vi "Dashboard Main.vi"() -> ()   [LabVIEW 2016]
uses:
  <vilib>/Utility/miscctls.llb/LVRowAndColumnTypeDef.ctl
  <vilib>/event_ctls.llb/eventvkey.ctl
  <vilib>/Rock Robotics/Network Tables/NT Read Numeric Array.vi
  <vilib>/Rock Robotics/WPI/Dashboard/WPI_DashboardLogging Global.vi
  <vilib>/Instr/_visa.llb/VISA Configure Serial Port (Instr).vi
panel:
  in  "Camera Settings Right":T1={"Frame Rate"=30, "Compression"=30, "Size"=1, "DB Camera Config"=FALSE} {"Frame Rate" scale=1.0..30.0; "Compression" scale=100.0..-1.0; "Size" items=["640x480", "320x240", "160x120"]}
  in  "Camera Name Right":string(combo)="No Camera Selection"
  out "Camera Info":cluster{"Mbps LED":bool, "Mbps":dbl, "fps":dbl} {"fps" format="%#.1g"; "Mbps" format="%#.1g"}
  in  "Camera Settings":T1={"Frame Rate"=30, "Compression"=30, "Size"=1, "DB Camera Config"=FALSE} {"Frame Rate" scale=1.0..30.0; "Compression" scale=100.0..-1.0; "Size" items=["640x480", "320x240", "160x120"]}
  in  "TCP":refnum<k5>
  in  "Rec Mode":enum32{"Stop", "Record", "Playback"}(radio)
  out "Robot IP":string
  out "Image Message":string="Timeout in Camera Communications"
  in  "Dashboard Tab":T2(tab)
  in  "Select Auto":string(combo)="Select Autonomous ..."
  out "NT Connection":bool
  out "MotorChart R":cluster{"Numeric":dbl, "Numeric":dbl}(graph)
  out "MotorChart L":cluster{"Numeric":dbl, "Numeric":dbl}(graph)
  out "MotorSliders R":cluster{"MotorSlide1":dbl, "MotorSlide2":dbl} {"MotorSlide2" scale=-1.0..1.0 scale format="%#_2e"; "MotorSlide1" scale=-1.0..1.0 scale format="%#_2e"}
  out "MotorSliders L":cluster{"MotorSlide1":dbl, "MotorSlide2":dbl} {"MotorSlide2" scale=-1.0..1.0 scale format="%#_2e"; "MotorSlide1" scale=-1.0..1.0 scale format="%#_2e"}
  out "Gyro":dbl(knob) scale=0.0..360.0
  out "JS1 Z":dbl(slide) scale=-1.0..1.0 scale format="%#_2e"
  out "JS1 Graph":cluster{"X":dbl, "Y":dbl}[](graph)
  out "JS1 Buttons":T3
  out "JS2 Z":dbl(slide) scale=-1.0..1.0 scale format="%#_2e"
  out "JS2 Graph":cluster{"X":dbl, "Y":dbl}[](graph)
  out "JS2 Buttons":T3
  out "Mode":T4(ring)=enum."Auto Disabled"
  out "read buffer":string
  out "Camera Image Right":T5(plugin-control)
  in  "DB/String 9":string
  in  "DB/String 8":string
  in  "DB/String 7":string
  in  "DB/String 6":string
  in  "DB/String 5":string
  in  "DB/String 4":string
  in  "DB/String 3":string
  in  "DB/String 2":string
  in  "DB/String 1":string
  in  "DB/String 0":string
  in  "DB/Slider 0":dbl(slide) scale=0.0..5.0
  in  "DB/Slider 1":dbl(slide) scale=0.0..5.0
  in  "DB/Slider 2":dbl(slide) scale=0.0..5.0
  in  "DB/Slider 3":dbl(slide) scale=0.0..5.0
  out "DB/LED 3":bool
  out "DB/LED 2":bool
  out "DB/LED 1":bool
  out "DB/LED 0":bool
  in  "DB/Button 3":bool
  in  "DB/Button 2":bool
  in  "DB/Button 1":bool
  in  "DB/Button 0":bool caption="New Name"
  in  "Test Slider":dbl(slide) scale=0.0..100.0 scale format="%#_3g"
  in  "On/Off":bool caption="Solenoid"
  in  "Test Name":u16(ring) items=["Select the test to run..."]
  in  "Test Tree":string(tree)
  in  "Motor":cluster{"Value":dbl, "Enable":bool} {"Value" scale=-1.0..1.0 scale format="%#_3g"}
  out "Progress":T6 {"Test Progress" scale=0.0..100.0}
  in  "Rev/Fwd":cluster{"Forward":bool, "Reverse":bool}
  in  "Test Ring":u16(ring) items=["Monochrome", "Color"]
  out "Cmd Status":string
  in  "Execute Command":bool
  in  "Command Params":string[][](table)
  in  "Command Selection":i32(listbox)
  in  "CheckList":i32(listbox)
  out "Tree":string(tree)
  out "Camera Image":T5(plugin-control)
  out "Background":bool
  in  "Camera Name":string(combo)="No Camera Selection"
  # "HW"
  # "HW"
  # "Joysticks"
  # "Drive Motors"
  # "Front"
  # "Right"
  # "Left"
  # "Back"
  # "This tab is a great place for autonomous settings and robot-specific values.\nPlace controls and indicators inside this tab and match name to\nDashboard Variables on robot. You can also delete this comment."
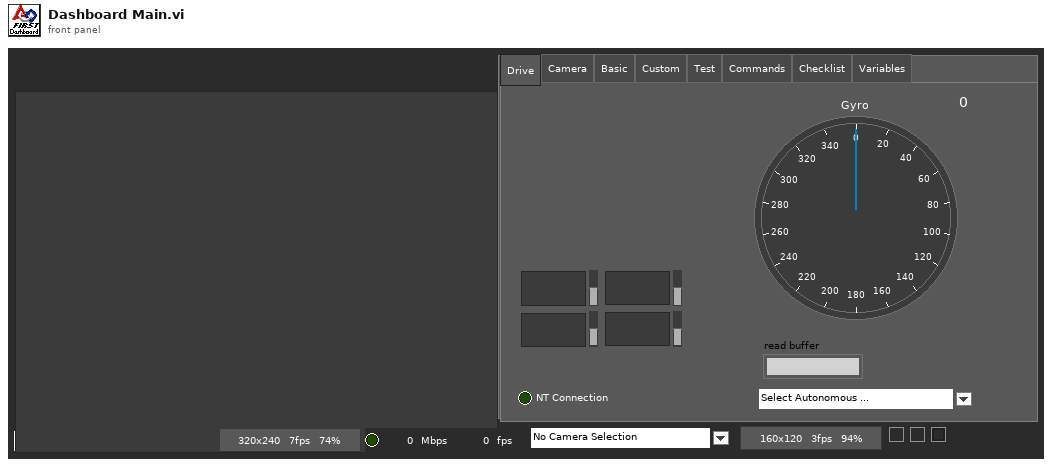
[diagram p1: front panel]
types:
  T1 = cluster{"Frame Rate":i32, "Compression":i32, "Size":u16, "DB Camera Config":bool}
  T2 = enum32{"Drive", "Camera", "Basic", "Custom", "Test", "Commands", "Checklist", "Variables"}
  T3 = cluster{bool, bool, bool, bool, bool, bool, bool, bool, bool, bool, bool, bool}
  T4 = enum8{"Tele-Op Disabled", "Tele-Op Enabled", "Auto Disabled", "Auto Enabled", "Test Disabled", "Test Enabled", "Disconnected", "No Code", "E-Stop"}
  T5 = typedef "IMAQ Image.ctl" = refnum<image>
  T6 = cluster{"Test Progress":u8, "Test Progress Text":string}
  T7 = typedef "Image Type" = u32
  T8 = cluster{"IDs":cluster{"RPC field ID":u16, "Unique ID":u16}, "String":string}
  T9 = enum32{"Drive", "Basic", "Custom", "Test", "Checklist", "Variables"}
  T10 = cluster{"Error Strings":string, "Disable Counts":cluster{u16, u16}, "Rail Faults":cluster{u16, u16, u16}, "Robot IP":string, "DB Mode":u8, "Event Info":cluster{"Name":string, "Type":u8, "Number":u16, "Replay":u8}}
  T11 = cluster{"Storage":cluster{"Disk Free":u64, "RAM Block":u32, "RAM free":u32}, "CPU Utilization":cluster{"CPU % ISR":sgl, "CPU % Time Crit":sgl, "CPU % Timed Str":sgl, "CPU % High":sgl, "CPU % Above":sgl, "CPU % Normal":sgl, "CPU % Low":sgl}, "CAN":cluster{"% Bus Utilization":sgl, "Bus Off Cnt":u32, "TX_FIFO Full Cnt":u32, "Receive Error Cnt":u8, "Transmit Error Cnt":u8}, "HID":cluster{"HID Outputs":u32, "Rumble Low":u16, "Rumble High":u16}[]}
  T12 = cluster{"Status bits":cluster{"Test Mode":bool, "Autonomous":bool, "Enabled":bool, "Code Start":bool, "Brownout":bool, "Reserved 2":bool, "Reserved 3":bool, "E-Stop":bool}, "Code Trace":cluster{"Disabled":bool, "TeleOp":bool, "Auto":bool, "Test":bool}, "Controller Type":enum16{"unknown", "cRIO", "roboRio"}, "Code?":enum16{"unknown", "noCode", "code"}, "Battery V":dbl}
  T13 = cluster{"Control Bits":cluster{"TestMode":bool, "Autonomous":bool, "Enabled":bool, "FMS Present":bool, bool, bool, bool, "E-Stop":bool}, "Team Station ":u8, "Countdown":sgl, "Joystick Values":cluster{"Axes":dbl[], "Buttons":bool[], "POVs":i16[]}[]}
  T14 = cluster{"Axes":dbl[], "Buttons":bool[], "POVs":i16[]}[]
  T15 = cluster{"Axes":dbl[], "Buttons":bool[], "POVs":i16[]}
  T16 = cluster{"Buttons[0]":bool, "Buttons[1]":bool, "Buttons[2]":bool, "Buttons[3]":bool, "Buttons[4]":bool, "Buttons[5]":bool, "Buttons[6]":bool, "Buttons[7]":bool, "Buttons[8]":bool, "Buttons[9]":bool, "Buttons[10]":bool, "Buttons[11]":bool}
  T17 = cluster{"Camera Image":refnum<vi>, "Dashboard Tab":refnum<vi>, "Background":refnum<vi>, "Rec Mode":refnum<vi>, "Test Slider":refnum<vi>, "On/Off ":refnum<vi>, "Test Ring":refnum<vi>, "Rev/Fwd":refnum<vi>, "Test Name":refnum<vi>, "Motor":refnum<vi>, "Progress":refnum<vi>, "CheckList":refnum<vi>, "Tree":refnum<vi>, "Test Tree":refnum<vi>, "Command Params":refnum<vi>, "Command Selection":refnum<vi>, "Execute Command":refnum<vi>, "Cmd Status":refnum<vi>, "Camera Settings":refnum<vi>, "Camera Name":refnum<vi>, "Camera Info":refnum<vi>, "Camera Settings Right":refnum<vi>, "Camera Name Right":refnum<vi>, "Camera Image Right":refnum<vi>}
  T18 = cluster{"Operation":enum16{"Update", "Clear"}, "Color Box":u32}[]
  T19 = typedef "eventvkey.ctl" = enum16{"ASCII", "Enter", "Return", "Shift", "Ctrl", "Alt", "Cmd", "Opt", "Caps", "NumLock", "Clear", "Break", "Up", "Down", "Left", "Right", "Insert", "Delete", "Home", "End", "PageUp", "PageDown", "Escape", "Help", "Pause", "ScrollLock", "F1", "F2", "F3", "F4", "F5", "F6", "F7", "F8", "F9", "F10", "F11", "F12", "F13", "F14", "F15", "F16", "F17", "F18", "F19", "F20", "F21", "F22", "F23", "F24", "Play", "VolumeUp", "VolumeDown", "Mute", "Two Byte Char"}
  T20 = cluster{"Image Size":bool, "Image Type":bool, "Pixel Value":bool, "ROI Information":bool, "Zoom Factor":bool}
  T21 = cluster{"Operation":enum16{"Update", "Clear"}, "Color Box":u32}
  T22 = typedef "LVRowAndColumnTypeDef.ctl" = cluster{"Row":i32, "Column":i32}
  T23 = cluster{"Shift":bool, "Ctrl":bool, "Alt":bool, "Cmd":bool, "Opt":bool}
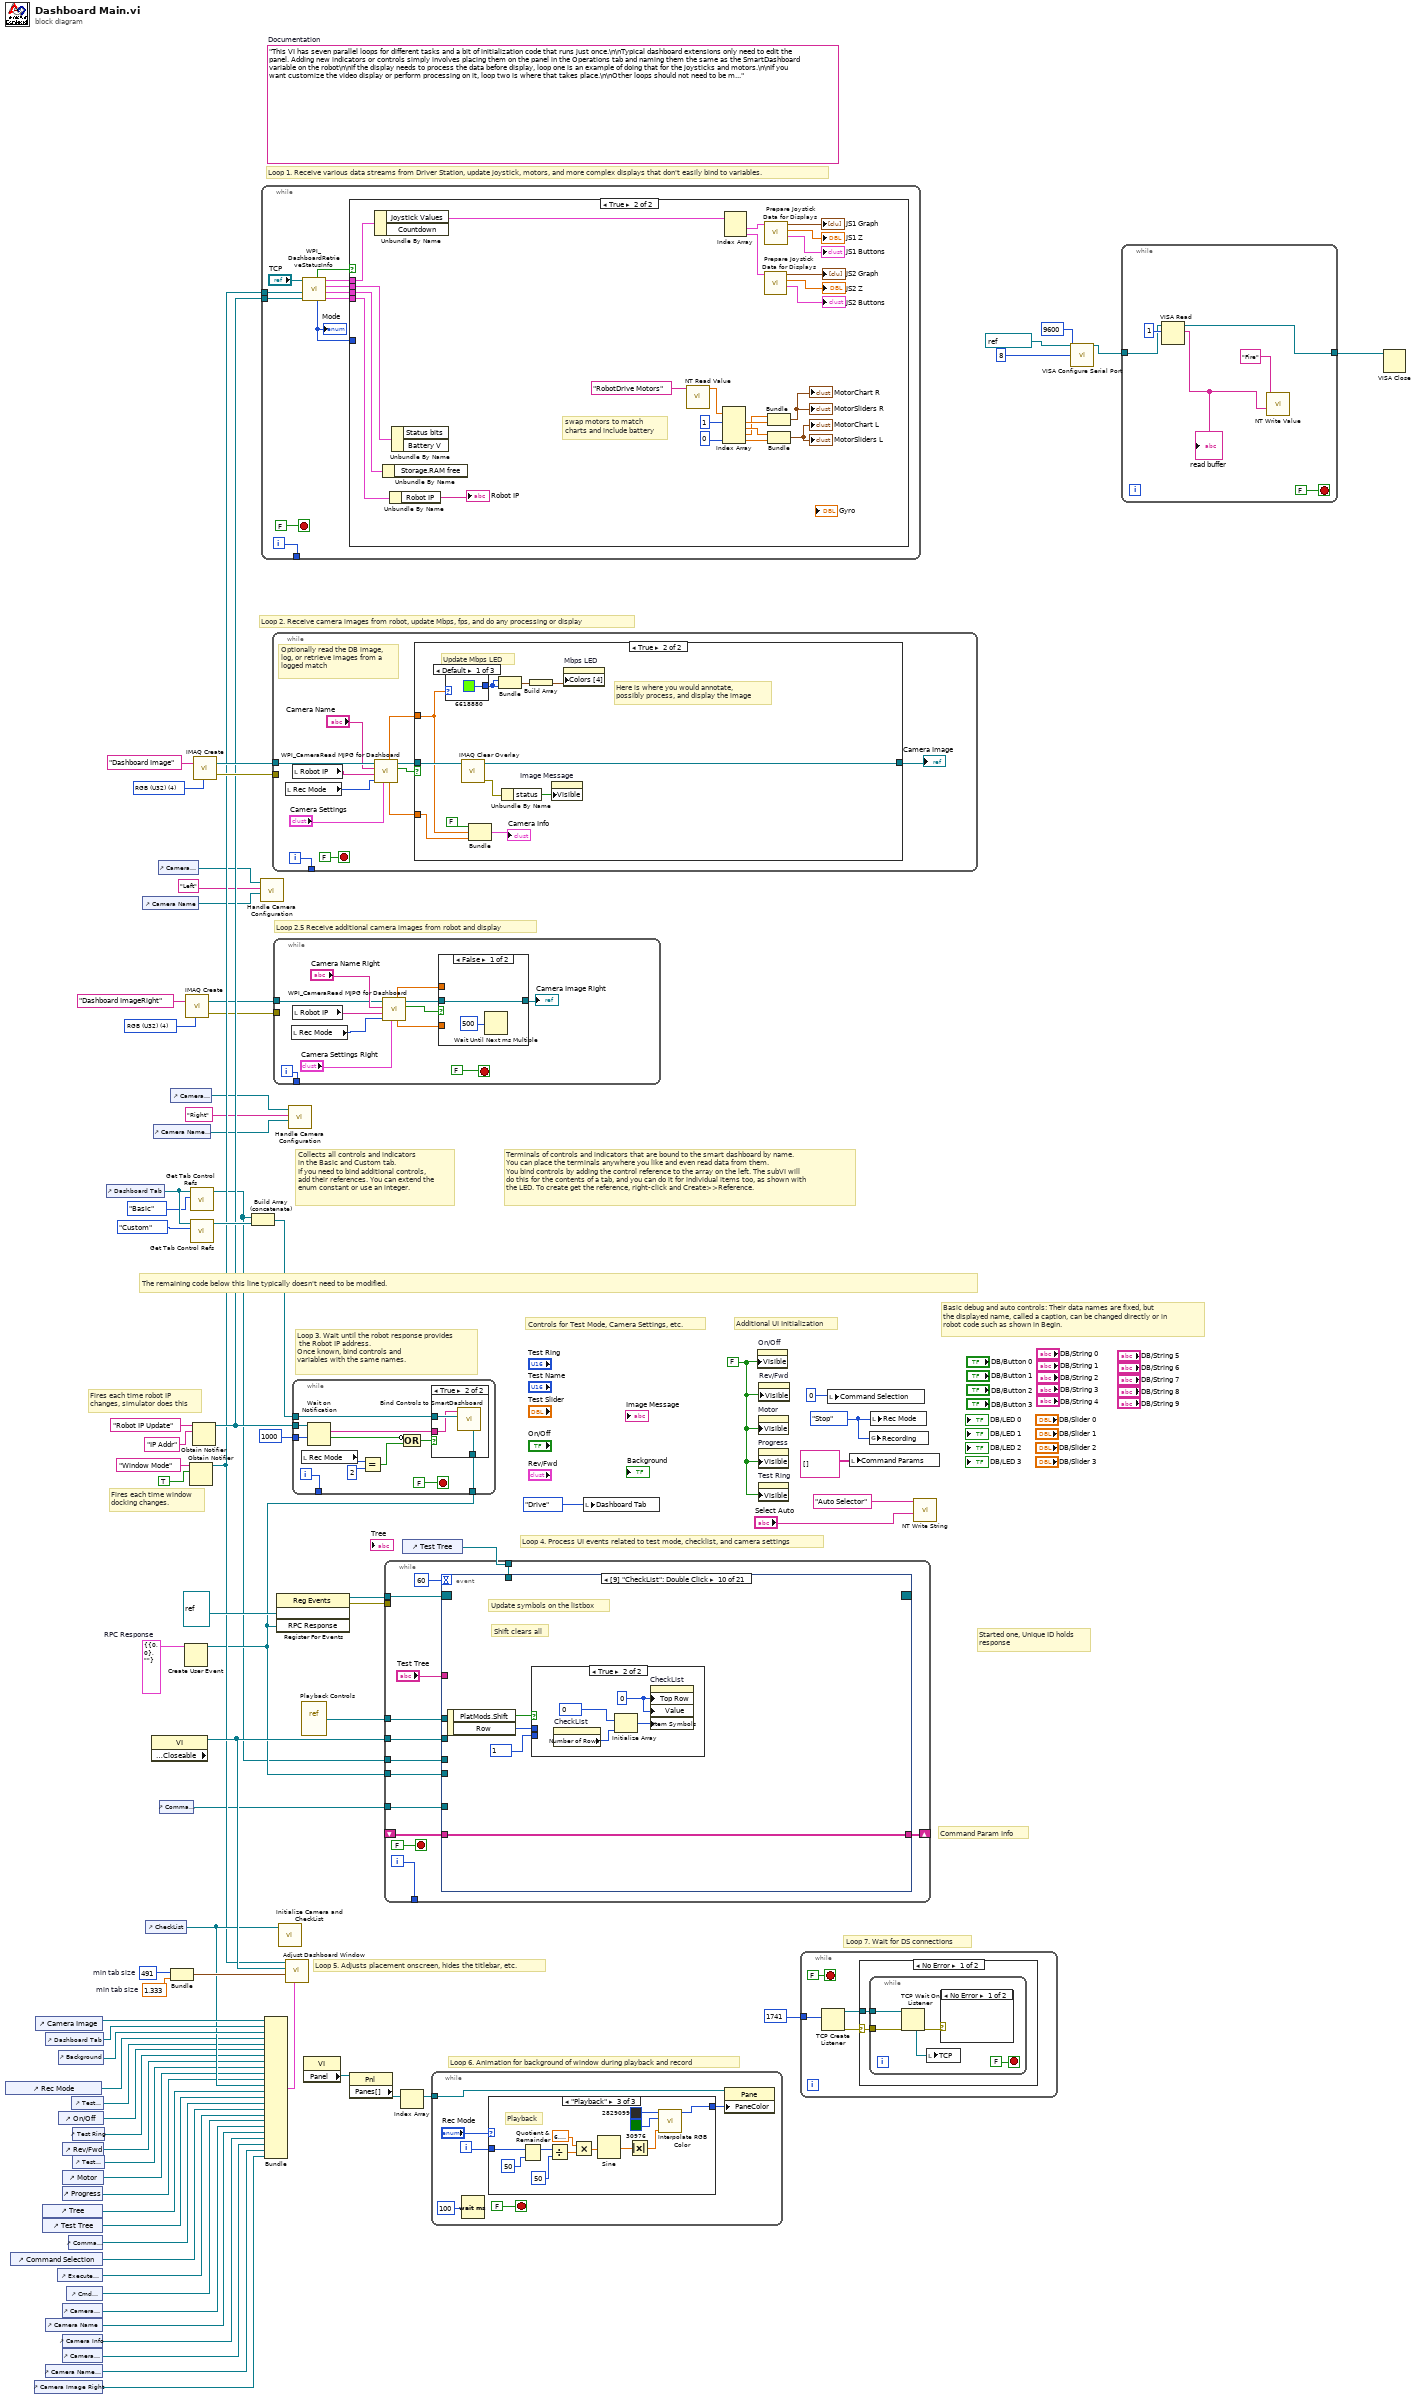
[diagram p0: block diagram]
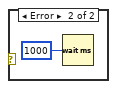
[diagram p3: hidden frame]
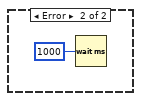
[diagram p4: hidden frame]
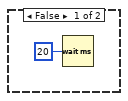
[diagram p5: hidden frame]
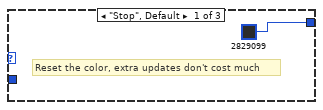
[diagram p6: hidden frame]
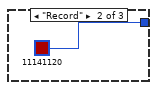
[diagram p7: hidden frame]
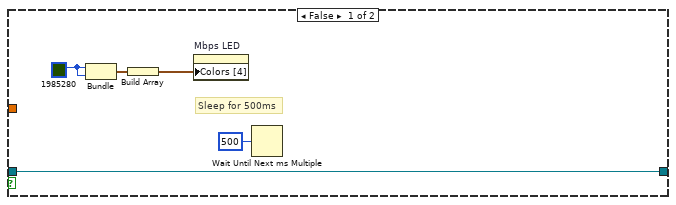
[diagram p9: hidden frame]
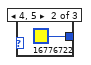
[diagram p10: hidden frame]
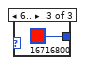
[diagram p11: hidden frame]
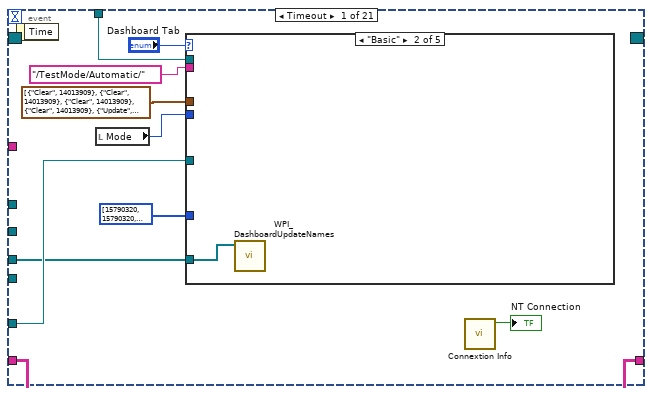
[diagram p12: hidden frame]
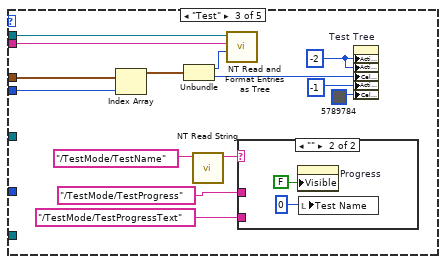
[diagram p14: hidden frame]
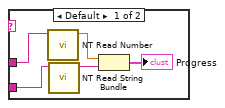
[diagram p15: hidden frame]
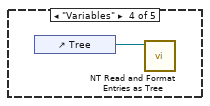
[diagram p16: hidden frame]
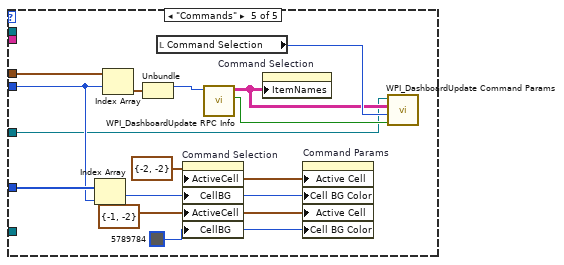
[diagram p17: hidden frame]
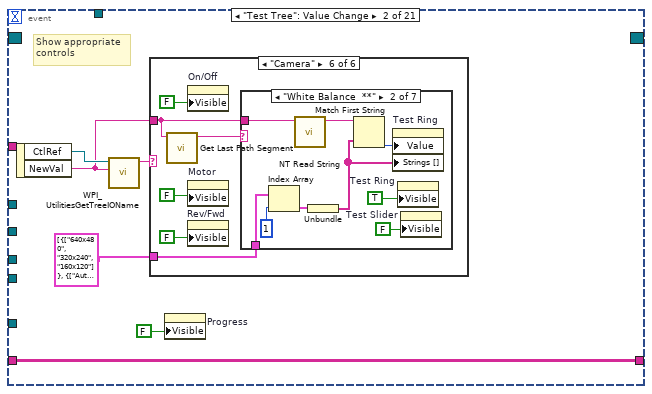
[diagram p18: hidden frame]
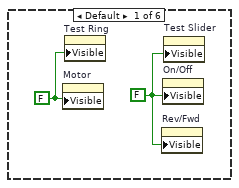
[diagram p19: hidden frame]
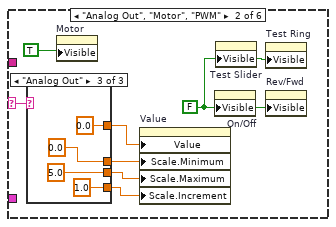
[diagram p20: hidden frame]
diagram:
  w15 = T7 4 items=["Grayscale (U8)", "Grayscale (I16)", "Grayscale (SGL)", "Complex (CSG)", "RGB (U32)", "HSL (U32)", "RGB (U64)"] ("Image Type")
  w31 = T8 {"IDs"={"RPC field ID"=0, "Unique ID"=0}, "String"=""}  # RPC Response
  w56 = 491  # min tab size
  w55 = 1.333  # min tab size
  w63 = enum32{"Stop", "Record", "Playback"}."Stop" ("Rec Mode")
  w38 = FALSE ("Visible")
  (unwired) "This VI has seven parallel loops for different tasks and a bit of initialization code that runs just once.\n\nTypical dashboard extensions only need to edit the panel. Adding new indicators or controls simply involves placing them on the panel in the Operations tab and naming them the same as the SmartDashboard variable on the robot\n\nIf the display needs to process the data before display, loop one is an example of doing that for the joysticks and motors.\n\nIf you want customize the video display or perform processing on it, loop two is where that takes place.\n\nOther loops should not need to be modified. They are pretty standard, and document the task they perform."  # Documentation
  w80 = T7 4 items=["Grayscale (U8)", "Grayscale (I16)", "Grayscale (SGL)", "Complex (CSG)", "RGB (U32)", "HSL (U32)", "RGB (U64)"] ("Image Type")
  # "Loop 2.5 Receive additional camera images from robot and display"
  # "Command Param Info"
  # "Started one, Unique ID holds\nresponse"
  # "Loop 7. Wait for DS connections"
  # "Basic debug and auto controls: Their data names are fixed, but\nthe displayed name, called a caption, can be changed directly or in\nrobot code such as shown in Begin."
  # "Controls for Test Mode, Camera Settings, etc."
  # "Additional UI Initialization"
  # "Loop 6. Animation for background of window during playback and record"
  # "Fires each time robot IP\nchanges, simulator does this"
  # "Fires each time window\ndocking changes."
  # "Collects all controls and indicators\nin the Basic and Custom tab.\nIf you need to bind additional controls,\nadd their references. You can extend the\nenum constant or use an integer."
  # "The remaining code below this line typically doesn't need to be modified."
  # "Loop 4. Process UI events related to test mode, checklist, and camera settings"
  # "Terminals of controls and indicators that are bound to the smart dashboard by name.\nYou can place the terminals anywhere you like and even read data from them.\nYou bind controls by adding the control reference to the array on the left. The subVI will\ndo this for the contents of a tab, and you can do it for individual items too, as shown with\nthe LED. To create get the reference, right-click and Create>>Reference."
  # "Loop 3. Wait until the robot response provides\n the Robot IP address.\nOnce known, bind controls and\nvariables with the same names."
  # "Loop 5. Adjusts placement onscreen, hides the titlebar, etc."
  # "Loop 1. Receive various data streams from Driver Station, update joystick, motors, and more complex displays that don't easily bind to variables."
  # "Loop 2. Receive camera images from robot, update Mbps, fps, and do any processing or display"
  n1 = control-ref of="Rec Mode"() -> (w44:refnum<vi>)
  n2 = control-ref of="Command Selection"() -> (w30:refnum<vi>)
  n3 = control-ref of="Camera Image Right"() -> (w6:refnum<vi>)
  n4 = control-ref of="Camera Image"() -> (w58:refnum<vi>)
  n5 = control-ref of="Tree"() -> (w48:refnum<vi>)
  n6 = control-ref of="Test Tree"() -> (w47:refnum<vi>)
  n7 = control-ref of="Dashboard Tab"() -> (w57:refnum<vi>)
  n8 = control-ref of="Camera Name"() -> (w21:refnum<vi>)
  n9 = control-ref of="Camera Name Right"() -> (w7:refnum<vi>)
  n10 = control-ref of="Execute Command"() -> (w32:refnum<vi>)
  n11 = control-ref of="Background"() -> (w53:refnum<vi>)
  n12 = control-ref of="On/Off"() -> (w42:refnum<vi>)
  n13 = control-ref of="Progress"() -> (w39:refnum<vi>)
  n14 = control-ref of="Camera Settings"() -> (w22:refnum<vi>)
  n15 = control-ref of="Camera Info"() -> (w20:refnum<vi>)
  n16 = control-ref of="Camera Settings Right"() -> (w8:refnum<vi>)
  n17 = control-ref of="Rev/Fwd"() -> (w40:refnum<vi>)
  n18 = control-ref of="Motor"() -> (w45:refnum<vi>)
  n19 = control-ref of="Cmd Status"() -> (w26:refnum<vi>)
  n20 = control-ref of="Command Params"() -> (w33:refnum<vi>)
  n21 = control-ref of="Test Slider"() -> (w43:refnum<vi>)
  n22 = control-ref of="Test Ring"() -> (w41:refnum<vi>)
  n23 = control-ref of="Test Name"() -> (w46:refnum<vi>)
  n24 = control-ref of="Dashboard Tab"() -> (w61:refnum<vi>)
  n25 = control-ref of="Camera Name"() -> (w23:refnum<vi>)
  n26 = control-ref of="CheckList"() -> (w49:refnum<vi>)
  n27 = property class="VI" props=["Front Panel.Closeable"]() -> (reference out=w62:refnum<vi>)  [unwired: 2 in, 2 out]
  n28 = control-ref of="Camera Name Right"() -> (w11:refnum<vi>)
  n29 = control-ref of="Camera Settings"() -> (w24:refnum<vi>)
  n30 = control-ref of="Command Params"() -> (w25:refnum<vi>)
  n31 = control-ref of="Camera Settings Right"() -> (w12:refnum<vi>)
  n32 = Bundle("min tab size"=w56, "min tab size"=w55) -> (w54:cluster{"min tab size":i32, "min tab size":dbl})  [unwired: 1 in]
  n33 = Create User Event(user event datatype=w31) -> (user event=w27:refnum<user-event>)  [unwired: 1 in, 1 out]
  n34 = call "IMAQ Create"("Image Name"="Dashboard ImageRight", "Image Type"=w15) -> ("New Image"=w14:T5, "error out"=w13:errorcluster)  [unwired: 2 in, 1 out]
  n35 = Obtain Notifier(name (unnamed)="Window Mode", notification data type=TRUE) -> (notifier out=w36:refnum<notifier>)  [unwired: 2 in, 2 out]
  n36 = call <vilib>:"Get Tab Control Refs.vi"("Page Index"=T9."Basic" ("Dashboard Tab"), "TabControl in"=w61) -> ("ControlsOnPage"=w19:refnum<vi>[])  [unwired: 9 in]
  n37 = call <vilib>:"Get Tab Control Refs.vi"("Page Index"=T9."Custom" ("Dashboard Tab"), "TabControl in"=w61) -> ("ControlsOnPage"=w60:refnum<vi>[])  [unwired: 9 in]
  n38 = Obtain Notifier(name (unnamed)="Robot IP Update", notification data type="IP Addr" ("name (unnamed)")) -> (notifier out=w37:refnum<notifier>)  [unwired: 2 in, 2 out]
  n39 = call "IMAQ Create"("Image Name"="Dashboard Image", "Image Type"=w80) -> ("New Image"=w78:T5, "error out"=w77:errorcluster)  [unwired: 2 in, 1 out]
  n40 = Build Array (concatenate)(w19, w60) -> (w59:refnum<vi>[])
  n41 = call "Handle Camera Configuration.vi"("CameraNameRef"=w23, "Camera File Name"="Left", "ClusterRef"=w24) -> ()  [unwired: 9 in]
  n42 = while {
    tunnel: [w90] -> _
    tunnel: w37 -> [w84]
    tunnel: w36 -> [w81]
    i -> [w90]
    stop <- FALSE stop-if-true
    n43 = call <vilib>:"WPI_DashboardRetrieveStatusInfo.vi"("Binding Refnum"=w84, "Window Mode Notifier"=w81, "TCP Cnx"="TCP") -> ("Power and Errors"=w85:T10, "Robot Metrics"=w88:T11, "Status Info"=w89:T12, "Control Info"=w86:T13, "Robot Mode"=w83:T4, "Process?"=w87:bool)  [unwired: 3 in]
    "Mode" <- w83
    n44 = case shown="True" w87 {
      tunnel: w89 -> [_ w116]
      tunnel: w88 -> [_ w115]
      tunnel: w86 -> [_ w114]
      tunnel: w85 -> [_ w113]
      tunnel: w83 -> [_ _]
      frame False {
        n45 = Wait (ms)(milliseconds to wait=u32 20) -> ()  [unwired: 1 out]
      }
      frame True {
        # "swap motors to match\ncharts and include battery"
        n46 = Unbundle By Name(w114) -> ("Joystick Values"=w104:T14)  [unwired: 1 out]
        n47 = Unbundle By Name(w115) -> ()  [unwired: 1 out]
        n48 = Unbundle By Name(w113) -> ("Robot IP"=→"Robot IP":string)
        n49 = Unbundle By Name(w116) -> ()  [unwired: 2 out]
        n50 = call-poly <vilib>:"NT Read Value.vi"("Name"="RobotDrive Motors") -> ("Numeric Array"=w94:dbl[])  [unwired: 9 in, 1 out]
        n51 = Index Array(array=w94, index #1=1, index #4=0) -> (element #1=w108:dbl, element #2=w109:dbl, element #3=w107:dbl, element #4=w112:dbl)  [unwired: 2 in]
        n52 = Index Array(array=w104) -> (element #1=w103:T15, element #2=w99:T15)  [unwired: 2 in]
        n53 = call "Prepare Joystick Data for Displays.vi"("Joystick Values"=w99) -> ("Buttons"=→"JS2 Buttons":T16, "Z Axis"=→"JS2 Z":dbl, "Cartesian Data"=→"JS2 Graph":cluster{"X axis":dbl, "X axis":dbl}[])  [unwired: 8 in]
        n54 = call "Prepare Joystick Data for Displays.vi"("Joystick Values"=w103) -> ("Buttons"=→"JS1 Buttons":T16, "Z Axis"=→"JS1 Z":dbl, "Cartesian Data"=→"JS1 Graph":cluster{"X axis":dbl, "X axis":dbl}[])  [unwired: 8 in]
        n55 = Bundle("Numeric"=w107, "Numeric"=w108) -> (→"MotorChart R" →"MotorSliders R":cluster{"Numeric":dbl, "Numeric":dbl})  [unwired: 1 in]
        n56 = Bundle("Numeric"=w109, "Numeric"=w112) -> (→"MotorChart L" →"MotorSliders L":cluster{"Numeric":dbl, "Numeric":dbl})  [unwired: 1 in]
      }
    }
  }
  n57 = Bundle("Camera Image"=w58, "Dashboard Tab"=w57, "Background"=w53, "Rec Mode"=w44, "Test Slider"=w43, "On/Off"=w42, "Test Ring"=w41, "Rev/Fwd"=w40, "Test Name"=w46, "Motor"=w45, "Progress"=w39, "CheckList"=w49, "Tree"=w48, "Test Tree"=w47, "Command Params"=w33, "Command Selection"=w30, "Execute Command"=w32, "Cmd Status"=w26, "Camera Settings"=w22, "Camera Name"=w21, "Camera Info"=w20, "Camera Settings Right"=w8, "Camera Name Right"=w7, "Camera Image Right"=w6) -> (w50:T17)  [unwired: 1 in]
  n58 = while {
    tunnel: w78 -> [w126]
    tunnel: w77 -> [_]
    tunnel: [w127] -> _
    i -> [w127]
    stop <- FALSE stop-if-true
    # "Optionally read the DB image,\nlog, or retrieve images from a\nlogged match"
    n59 = local read "Rec Mode"() -> (w122:enum32{"Stop", "Record", "Playback"})
    n60 = local read "Robot IP"() -> (w121:string)
    n61 = call <vilib>:"WPI_CameraRead MJPG for Dashboard.vi"("Camera Settings"="Camera Settings", "Rec Mode"=w122, "Robot IP"=w121, "Camera Name"="Camera Name", "Refnum in"=w126) -> ("Active"=w124:bool, "Refnum out"=w125:T5, "FPS"=w123:dbl, "Bandwidth (Mbps)"=w120:dbl)  [unwired: 3 in]
    n62 = case shown="True" w124 {
      tunnel: w125 -> [w129 w140]
      tunnel: w120 -> [_ w137]
      tunnel: w123 -> [_ w138]
      tunnel: [w129 w134] -> w117
      frame False {
        w131 = u32 1985280 ("Color Box")
        # "Sleep for 500ms"
        n63 = Bundle("Color Box"=w131, "Color Box"=w131) -> (w132:cluster{"Color Box":u32, "Color Box":u32})  [unwired: 1 out]
        n64 = Build Array(w132) -> (w130:cluster{"Color Box":u32, "Color Box":u32}[])
        n65 = property on="Mbps LED" class="Bool (strict)"("Colors [4]"=w130) -> ()  [unwired: 2 in, 2 out]
        n66 = Wait Until Next ms Multiple(millisecond multiple=u32 500) -> ()  [unwired: 1 out]
      }
      frame True {
        # "Here is where you would annotate,\npossibly process, and display the image"
        # "Update Mbps LED"
        n67 = case shown="Default" w137 {
          tunnel: [u32 6618880 ("Color Box") u32 16776722 ("Color Box") u32 16716800 ("Color Box")] -> w141
          frame Default {
          }
          frame 4, 5 {
          }
          frame 6.. {
          }
        }
        n68 = call "IMAQ Clear Overlay"("Image"=w140) -> ("error out"=w143:errorcluster, "Image Out"=w134:T5)  [unwired: 2 in, 7 out]
        n69 = Bundle(FALSE, "Bandwidth (Mbps)"=w137, "FPS"=w138) -> (→"Camera Info":cluster{bool, "Bandwidth (Mbps)":dbl, "FPS":dbl})  [unwired: 1 in]
        n70 = Bundle("Color Box"=w141, "Color Box"=w141) -> (w142:cluster{"Color Box":u32, "Color Box":u32})  [unwired: 1 out]
        n71 = Unbundle By Name(w143) -> ("status"=w144:bool)
        n72 = Build Array(w142) -> (w139:cluster{"Color Box":u32, "Color Box":u32}[])
        n73 = property on="Image Message" class="Str"("Visible"=w144) -> ()  [unwired: 2 in, 2 out]
        n74 = property on="Mbps LED" class="Bool (strict)"("Colors [4]"=w139) -> ()  [unwired: 2 in, 2 out]
      }
    }
    "Camera Image" <- w117
  }
  n75 = while {
    tunnel: w14 -> [w158]
    tunnel: w13 -> [_]
    tunnel: [w152] -> _
    i -> [w152]
    stop <- FALSE stop-if-true
    n76 = local read "Rec Mode"() -> (w156:enum32{"Stop", "Record", "Playback"})
    n77 = local read "Robot IP"() -> (w157:string)
    n78 = call <vilib>:"WPI_CameraRead MJPG for Dashboard.vi"("Camera Settings"="Camera Settings Right", "Rec Mode"=w156, "Robot IP"=w157, "Camera Name"="Camera Name Right", "Refnum in"=w158) -> ("Active"=w151:bool, "Refnum out"=w154:T5, "FPS"=w149:dbl, "Bandwidth (Mbps)"=w150:dbl)  [unwired: 3 in]
    n79 = case shown="False" w151 {
      tunnel: w154 -> [w160 w162]
      tunnel: w150 -> [_ _]
      tunnel: w149 -> [_ _]
      tunnel: [w160 w162] -> w148
      frame False {
        n80 = Wait Until Next ms Multiple(millisecond multiple=u32 500) -> ()  [unwired: 1 out]
      }
      frame True {
      }
    }
    "Camera Image Right" <- w148
  }
  n81 = register-events(refnum<vi> refnum, w27) -> (reference out=w67:refnum<event-registration>, error out=w66:errorcluster)  [unwired: 2 in]
  n82 = call "Initialize Camera and CheckList.vi"("ListBox in"=w49) -> ()  [unwired: 11 in]
  n83 = call "Adjust Dashboard Window.vi"("Sizing Refnums"=w50, "Size Constraints"=w54, "VI"=w62, "WIn Mode"=w36) -> ()  [unwired: 8 in]
  n84 = call "Handle Camera Configuration.vi"("CameraNameRef"=w11, "Camera File Name"="Right", "ClusterRef"=w12) -> ()  [unwired: 9 in]
  n85 = while {
    tunnel: w59 -> [w174]
    tunnel: w37 -> [w172]
    tunnel: [w170] -> _
    tunnel: u32 1000 ("milliseconds to wait") -> [w169]
    tunnel: w27 -> [w163]
    i -> [w170]
    stop <- FALSE stop-if-true
    n86 = local read "Rec Mode"() -> (w165:enum32{"Stop", "Record", "Playback"})
    n87 = Wait on Notification(notifier=w172, timeout in ms (-1)=w169) -> (notification=w171:string, timed out?=w167:bool)  [unwired: 2 in, 2 out]
    n88 = Equal?(x=w165, y=u16 2 ("Rec Mode")) -> (x = y?=w166:bool)
    n89 = Compound Arithmetic op=OR(invert w167, w166) -> (w168:bool)
    n90 = case shown="True" w168 {
      tunnel: w174 -> [_ w177]
      tunnel: w171 -> [_ w176]
      tunnel: w163 -> [_ w175]
      frame False {
      }
      frame True {
        n91 = call <vilib>:"Bind Controls to SmartDashboard.vi"("RPC ref"=w175, "Bound Control Refs"=w177, "Server IP Address"=w176) -> ()  [unwired: 9 in]
      }
    }
  }
  n92 = vi-ref "Playback Controls.vi"() -> (w68:refnum<vi>)
  n93 = property class="VI"() -> ("Panel"=w70:refnum<vi>)  [unwired: 2 in, 2 out]
  n94 = property class="Pnl"(reference=w70) -> ("Panes[]"=w71:refnum<vi>[])  [unwired: 1 in, 2 out]
  n95 = Index Array(array=w71) -> (element=w69:refnum<vi>)  [unwired: 1 in]
  n96 = control-ref of="Test Tree"() -> (w72:refnum<vi>)
  n97 = while {
    tunnel: [w187] -> _
    tunnel: w72 -> [w186]
    tunnel: w68 -> [w185]
    tunnel: w67 -> [w184]
    tunnel: w66 -> [_]
    tunnel: w62 -> [w183]
    tunnel: w27 -> [w182]
    tunnel: w25 -> [w181]
    shift-right: [w180] -> _
    shift-left: _ -> [w179]
    tunnel: w19 -> [w178]
    i -> [w187]
    stop <- FALSE stop-if-true
    n98 = event shown="[9] \"CheckList\": Double Click" {
      selector: w184 -> [_ _ _ _ _ _ _ _ _ _ _ _ _ _ _ _ _ _ _ _ _]
      dyn-events: [_ _ _ _ _ _ _ _ _ _ _ _ _ _ _ _ w443 _ _ _ _] -> _
      timeout: u32 60 ("milliseconds to wait") -> [_ _ _ _ _ _ _ _ _ _ _ _ _ _ _ _ _ _ _ _ _]
      tunnel: w186 -> [w199 _ _ _ _ _ _ _ _ _ _ _ _ _ _ _ _ _ _ _ _]
      tunnel: "Test Tree" -> [_ _ _ _ _ _ _ _ _ _ _ w410 w418 w420 w424 w432 _ _ _ _ _]
      tunnel: w185 -> [_ _ _ _ _ _ _ _ _ _ _ _ _ _ _ _ w445 _ w463 _ _]
      tunnel: w183 -> [_ _ _ _ _ _ _ _ _ _ _ _ _ _ _ _ w441 _ _ _ _]
      tunnel: w182 -> [_ _ _ _ _ _ _ _ _ _ _ _ _ _ _ _ w437 _ _ _ _]
      tunnel: w181 -> [w194 _ _ _ _ _ w361 _ _ _ _ _ _ _ _ _ _ _ _ _ _]
      tunnel: [w193 w238 w340 w345 w354 w358 w359 w368 w378 w385 w397 w409 w416 w419 w423 w431 w436 w458 w460 w464 w475] -> w180
      tunnel: w179 -> [w193 w238 w340 w345 w354 w358 w359 _ _ w385 w397 w409 w416 w419 w423 w431 w436 w458 w460 w464 w475]
      tunnel: w178 -> [w191 _ _ _ _ _ _ _ _ _ _ _ _ _ _ _ _ _ _ _ _]
      event Timeout {
        n99 = event-data() -> ()  [unwired: 1 in, 1 out]
        n100 = local read "Mode"() -> (w196:T4)
        n101 = case shown="\"Basic\"" "Dashboard Tab" {
          tunnel: w199 -> [_ _ w215 _ _]
          tunnel: "/TestMode/Automatic/" ("Name Pattern") -> [_ _ w214 _ _]
          tunnel: T18 [{"Operation"=enum."Clear", "Color Box"=14013909}, {"Operation"=enum."Clear", "Color Box"=14013909}, {"Operation"=enum."Clear", "Color Box"=14013909}, {"Operation"=enum."Clear", "Color Box"=14013909}, {"Operation"=enum."Update", "Color Box"=14013909}, {"Operation"=enum."Update", "Color Box"=16777215}, {"Operation"=enum."Clear", "Color Box"=14013909}, {"Operation"=enum."Clear", "Color Box"=14013909}, {"Operation"=enum."Clear", "Color Box"=14013909}] -> [_ _ w207 _ w231]
          tunnel: w196 -> [_ _ w206 _ w230]
          tunnel: u32[] [15790320, 15790320, 15790320, 15790320, 16777215, 16777215, 15790320, 15790320, 15790320] -> [_ _ _ _ w236]
          tunnel: w194 -> [_ _ _ _ w224]
          tunnel: w191 -> [_ w201 _ _ _]
          frame "Custom", Default {
          }
          frame "Basic" {
            n102 = call <vilib>:"WPI_DashboardUpdateNames.vi"("Controls on Tab"=w201) -> ()  [unwired: 11 in]
          }
          frame "Test" {
            w213 = -2 ("Active Item:Row Number")
            n103 = Index Array(array=w207, index=w206) -> (element=w208:T21)
            n104 = Unbundle(w208) -> ("Operation"=w209:enum16{"Update", "Clear"}, "Color Box"=w210:u32)
            n105 = call <vilib>:"NT Read String.vi"("Name"="/TestMode/TestName") -> ("String"=w204:string)  [unwired: 9 in, 1 out]
            n106 = call <vilib>:"NT Read and Format Entries as Tree.vi"("Operation"=w209, "Name Pattern"=w214, "Tree Refnum"=w215) -> ()  [unwired: 7 in, 2 out]
            n107 = case shown="\"\"" w204 {
              tunnel: "/TestMode/TestProgress" ("Name") -> [w217 _]
              tunnel: "/TestMode/TestProgressText" ("Name") -> [w216 _]
              frame Default {
                n108 = call <vilib>:"NT Read Number.vi"("Name"=w217) -> ("Numeric"=w218:dbl)  [unwired: 9 in, 1 out]
                n109 = call <vilib>:"NT Read String.vi"("Name"=w216) -> ("String"=w219:string)  [unwired: 9 in, 1 out]
                n110 = Bundle("Numeric"=w218, "String"=w219) -> (→"Progress":cluster{"Numeric":dbl, "String":string})  [unwired: 1 in]
              }
              frame "" {
                n111 = property on="Progress" class="Clust (strict)"("Visible"=FALSE) -> ()  [unwired: 2 in, 2 out]
                n112 = local write "Test Name"(u16 0) -> ()
              }
            }
            n113 = property on="Test Tree" class="Tree (strict)"("Active Item Row Number"=w213, "ActiveColNum"=w213, "CellBG"=w210, "Active Item Row Number"=-1 ("Active Item:Row Number"), "CellBG"=u32 5789784 ("Color Box")) -> ()  [unwired: 2 in, 2 out]
          }
          frame "Variables" {
            n114 = control-ref of="Tree"() -> (w223:refnum<vi>)
            n115 = call <vilib>:"NT Read and Format Entries as Tree.vi"("Tree Refnum"=w223) -> ()  [unwired: 9 in, 2 out]
          }
          frame "Commands" {
            w232 = u32 5789784 ("Color Box")
            w233 = T22 {"Row"=-1, "Column"=-2} ("Active Cell:Active Cell")
            w235 = T22 {"Row"=-2, "Column"=-2} ("Active Cell:Active Cell")
            n116 = Index Array(array=w236, index=w230) -> (element=w234:u32)
            n117 = Index Array(array=w231, index=w230) -> (element=w229:T21)
            n118 = Unbundle(w229) -> ("Operation"=w228:enum16{"Update", "Clear"})  [unwired: 1 out]
            n119 = local read "Command Selection"() -> (w227:i32)
            n120 = property on="Command Selection" class="MCListbox (strict)"("ActiveCell"=w235, "CellBG"=w234, "ActiveCell"=w233, "CellBG"=w232) -> ()  [unwired: 2 in, 2 out]
            n121 = call <vilib>:"WPI_DashboardUpdate RPC Info.vi"("Operation"=w228) -> ("update"=w226:bool, "commands"=w225:string[][])  [unwired: 9 in]
            n122 = property on="Command Selection" class="MCListbox (strict)"("ItemNames"=w225) -> ()  [unwired: 2 in, 2 out]
            n123 = property on="Command Params" class="Tbl (strict)"("Active Cell"=w235, "Cell BG Color"=w234, "Active Cell"=w233, "Cell BG Color"=w232) -> ()  [unwired: 2 in, 2 out]
            n124 = call <vilib>:"WPI_DashboardUpdate Command Params.vi"("Update"=w226, "NewVal"=w227, "Commands"=w225, "Param Tbl"=w224) -> ()  [unwired: 7 in, 1 out]
          }
        }
        n125 = call <vilib>:"Connextion Info.vi"() -> ("Connected"=→"NT Connection":bool)  [unwired: 10 in, 1 out]
      }
      event "Test Tree": Value Change {
        # "Show appropriate\ncontrols"
        n126 = event-data() -> ("CtlRef"=w241:refnum<vi>, "NewVal"=w239:string)  [unwired: 1 in]
        n127 = call <vilib>:"WPI_UtilitiesGetTreeIOName.vi"("NewVal"=w239, "TreeControl in"=w241) -> ("I/O Name"=w242:string)  [unwired: 9 in]
        n128 = case shown="\"Camera\"" w242 {
          selector: w242 -> [_ w249 _ w271 w280 _]
          tunnel: w239 -> [_ _ w268 w270 _ w287]
          tunnel: cluster{string[]}[] [{["640x480", "320x240", "160x120"]}, {["Auto", "Fixed indoor", "Fixed outdoor 1", "Fixed outdoor 2", "Fixed fluorescent 1", "Fixed fluorescent 2", "Hold current"]}, {["Auto", "Flicker-free 50 Hz", "Flicker-free 60 Hz", "Hold current"]}, {["None", "Prioritize frame rate", "Prioritize image quality"]}, {["Monochrome", "Color"]}] -> [_ _ _ _ _ w286]
          frame Default {
            w244 = FALSE ("Visible")
            w243 = FALSE ("Visible")
            n129 = property on="Motor" class="Clust (strict)"("Visible"=w243) -> ()  [unwired: 2 in, 2 out]
            n130 = property on="Test Ring" class="Ring (strict)"("Visible"=w243) -> ()  [unwired: 2 in, 2 out]
            n131 = property on="Rev/Fwd" class="Clust (strict)"("Visible"=w244) -> ()  [unwired: 2 in, 2 out]
            n132 = property on="On/Off" class="Bool (strict)"("Visible"=w244) -> ()  [unwired: 2 in, 2 out]
            n133 = property on="Test Slider" class="Slide (strict)"("Visible"=w244) -> ()  [unwired: 2 in, 2 out]
          }
          frame "Analog Out", "Motor", "PWM" {
            w250 = FALSE ("Visible")
            n134 = case shown="\"Analog Out\"" w249 {
              tunnel: [1.0 ("Value") -1.0 ("Value") 0.0 ("Value")] -> w248
              tunnel: [255.0 ("Value") 1.0 ("Value") 5.0 ("Value")] -> w247
              tunnel: [128.0 ("Value") 0.0 ("Value") 0.0 ("Value")] -> w246
              tunnel: [64.0 ("Value") 0.5 ("Value") 1.0 ("Value")] -> w245
              frame "PWM" {
              }
              frame "Motor", Default {
              }
              frame "Analog Out" {
              }
            }
            n135 = property on="Motor" class="Clust (strict)"("Visible"=TRUE) -> ()  [unwired: 2 in, 2 out]
            n136 = property on="Value" class="Slide (strict)"("Value"=w246, "Scale.Minimum"=w248, "Scale.Maximum"=w247, "Scale.Increment"=w245) -> ()  [unwired: 2 in, 2 out]
            n137 = property on="On/Off" class="Bool (strict)"("Visible"=w250) -> ()  [unwired: 2 in, 2 out]
            n138 = property on="Test Slider" class="Slide (strict)"("Visible"=w250) -> ()  [unwired: 2 in, 2 out]
            n139 = property on="Test Ring" class="Ring (strict)"("Visible"=w250) -> ()  [unwired: 2 in, 2 out]
            n140 = property on="Rev/Fwd" class="Clust (strict)"("Visible"=w250) -> ()  [unwired: 2 in, 2 out]
          }
          frame "Servo" {
            w266 = FALSE ("Visible")
            n141 = call <vilib>:"NT Read Number.vi"("Name"=w268) -> ("Numeric"=w267:dbl)  [unwired: 9 in, 1 out]
            n142 = property on="Test Slider" class="Slide (strict)"("Visible"=TRUE, "Scale.Maximum"=170.0 ("Scale.Range:Maximum")) -> ()  [unwired: 2 in, 2 out]
            n143 = local write "Test Slider"(w267) -> ()
            n144 = property on="Motor" class="Clust (strict)"("Visible"=w266) -> ()  [unwired: 2 in, 2 out]
            n145 = property on="Rev/Fwd" class="Clust (strict)"("Visible"=w266) -> ()  [unwired: 2 in, 2 out]
            n146 = property on="On/Off" class="Bool (strict)"("Visible"=w266) -> ()  [unwired: 2 in, 2 out]
            n147 = property on="Test Ring" class="Ring (strict)"("Visible"=w266) -> ()  [unwired: 2 in, 2 out]
          }
          frame "Relay", "Solenoid" {
            w269 = FALSE ("Visible")
            n148 = property on="Motor" class="Clust (strict)"("Visible"=w269) -> ()  [unwired: 2 in, 2 out]
            n149 = property on="Test Slider" class="Slide (strict)"("Visible"=w269) -> ()  [unwired: 2 in, 2 out]
            n150 = Search and Replace String(input string=w270, search string="/Value  **", replace string="/Direction") -> (result string=w276:string)  [unwired: 5 in, 3 out]
            n151 = property on="Test Ring" class="Ring (strict)"("Visible"=w269) -> ()  [unwired: 2 in, 2 out]
            n152 = call <vilib>:"NT Read String.vi"("Name"=w276) -> ("String"=w274:string)  [unwired: 9 in, 1 out]
            n153 = Equal?(x="Both directions", y=w274) -> (x = y?=w272:bool)
            n154 = Not(x=w272) -> (.not. x?=w273:bool)
            n155 = property on="Rev/Fwd" class="Clust (strict)"("Visible"=w272) -> ()  [unwired: 2 in, 2 out]
            n156 = property on="On/Off" class="Bool (strict)"("Visible"=w273, "Caption.Text"=w271) -> ()  [unwired: 2 in, 2 out]
          }
          frame "Compressor", "Digital Out" {
            w279 = FALSE ("Visible")
            # "Get direction and finish"
            n157 = property on="Motor" class="Clust (strict)"("Visible"=w279) -> ()  [unwired: 2 in, 2 out]
            n158 = property on="Test Slider" class="Slide (strict)"("Visible"=w279) -> ()  [unwired: 2 in, 2 out]
            n159 = property on="Test Ring" class="Ring (strict)"("Visible"=w279) -> ()  [unwired: 2 in, 2 out]
            n160 = property on="On/Off" class="Bool (strict)"("Visible"=TRUE, "Caption.Text"=w280) -> ()  [unwired: 2 in, 2 out]
            n161 = property on="Rev/Fwd" class="Clust (strict)"("Visible"=FALSE) -> ()  [unwired: 2 in, 2 out]
          }
          frame "Camera" {
            n162 = call <vilib>:"Get Last Path Segment.vi"("String in"=w287) -> ("String out"=w288:string)  [unwired: 10 in]
            n163 = property on="On/Off" class="Bool (strict)"("Visible"=FALSE) -> ()  [unwired: 2 in, 2 out]
            n164 = property on="Motor" class="Clust (strict)"("Visible"=FALSE) -> ()  [unwired: 2 in, 2 out]
            n165 = property on="Rev/Fwd" class="Clust (strict)"("Visible"=FALSE) -> ()  [unwired: 2 in, 2 out]
            n166 = case shown="\"White Balance  **\"" w288 {
              tunnel: w287 -> [w294 w303 w312 w321 w330 _ w336]
              tunnel: w286 -> [w292 w300 w309 w318 w327 _ _]
              frame "Size  **" {
                n167 = Index Array(array=w292) -> (element=w291:cluster{string[]})  [unwired: 1 in]
                n168 = call <vilib>:"NT Read String.vi"("Name"=w294) -> ("String"=w293:string)  [unwired: 9 in, 1 out]
                n169 = Unbundle(w291) -> (w289:string[])
                n170 = Match First String(2:w289, 3:w293) -> (0:w290:i32)  [unwired: 1 out]
                n171 = property on="Test Ring" class="Ring (strict)"("Value"=w290, "Strings []"=w289) -> ()  [unwired: 2 in, 2 out]
                n172 = property on="Test Ring" class="Ring (strict)"("Visible"=TRUE) -> ()  [unwired: 2 in, 2 out]
                n173 = property on="Test Slider" class="Slide (strict)"("Visible"=FALSE) -> ()  [unwired: 2 in, 2 out]
              }
              frame "White Balance  **" {
                n174 = Index Array(array=w300, index=1) -> (element=w301:cluster{string[]})
                n175 = call <vilib>:"NT Read String.vi"("Name"=w303) -> ("String"=w302:string)  [unwired: 9 in, 1 out]
                n176 = Unbundle(w301) -> (w298:string[])
                n177 = Match First String(2:w298, 3:w302) -> (0:w297:i32)  [unwired: 1 out]
                n178 = property on="Test Ring" class="Ring (strict)"("Value"=w297, "Strings []"=w298) -> ()  [unwired: 2 in, 2 out]
                n179 = property on="Test Ring" class="Ring (strict)"("Visible"=TRUE) -> ()  [unwired: 2 in, 2 out]
                n180 = property on="Test Slider" class="Slide (strict)"("Visible"=FALSE) -> ()  [unwired: 2 in, 2 out]
              }
              frame "Exposure  **" {
                n181 = Index Array(array=w309, index=2) -> (element=w310:cluster{string[]})
                n182 = call <vilib>:"NT Read String.vi"("Name"=w312) -> ("String"=w311:string)  [unwired: 9 in, 1 out]
                n183 = Unbundle(w310) -> (w306:string[])
                n184 = Match First String(2:w306, 3:w311) -> (0:w307:i32)  [unwired: 1 out]
                n185 = property on="Test Ring" class="Ring (strict)"("Value"=w307, "Strings []"=w306) -> ()  [unwired: 2 in, 2 out]
                n186 = property on="Test Ring" class="Ring (strict)"("Visible"=TRUE) -> ()  [unwired: 2 in, 2 out]
                n187 = property on="Test Slider" class="Slide (strict)"("Visible"=FALSE) -> ()  [unwired: 2 in, 2 out]
              }
              frame "Exposure Priority  **" {
                n188 = Index Array(array=w318, index=3) -> (element=w319:cluster{string[]})
                n189 = call <vilib>:"NT Read String.vi"("Name"=w321) -> ("String"=w320:string)  [unwired: 9 in, 1 out]
                n190 = Unbundle(w319) -> (w315:string[])
                n191 = Match First String(2:w315, 3:w320) -> (0:w316:i32)  [unwired: 1 out]
                n192 = property on="Test Ring" class="Ring (strict)"("Value"=w316, "Strings []"=w315) -> ()  [unwired: 2 in, 2 out]
                n193 = property on="Test Ring" class="Ring (strict)"("Visible"=TRUE) -> ()  [unwired: 2 in, 2 out]
                n194 = property on="Test Slider" class="Slide (strict)"("Visible"=FALSE) -> ()  [unwired: 2 in, 2 out]
              }
              frame "Color Enable  **" {
                n195 = Index Array(array=w327, index=4) -> (element=w328:cluster{string[]})
                n196 = call <vilib>:"NT Read String.vi"("Name"=w330) -> ("String"=w329:string)  [unwired: 9 in, 1 out]
                n197 = Unbundle(w328) -> (w324:string[])
                n198 = Match First String(2:w324, 3:w329) -> (0:w325:i32)  [unwired: 1 out]
                n199 = property on="Test Ring" class="Ring (strict)"("Value"=w325, "Strings []"=w324) -> ()  [unwired: 2 in, 2 out]
                n200 = property on="Test Ring" class="Ring (strict)"("Visible"=TRUE) -> ()  [unwired: 2 in, 2 out]
                n201 = property on="Test Slider" class="Slide (strict)"("Visible"=FALSE) -> ()  [unwired: 2 in, 2 out]
              }
              frame Default {
                n202 = property on="Test Ring" class="Ring (strict)"("Visible"=FALSE) -> ()  [unwired: 2 in, 2 out]
                n203 = property on="Test Slider" class="Slide (strict)"("Visible"=FALSE) -> ()  [unwired: 2 in, 2 out]
              }
              frame "Brightness  **", "Color Level  **", "Compression  **", "FPS  **", "Sharpness  **" {
                n204 = call <vilib>:"NT Read Number.vi"("Name"=w336) -> ("Numeric"=w335:dbl)  [unwired: 9 in, 1 out]
                n205 = local write "Test Slider"(w335) -> ()
                n206 = property on="Test Slider" class="Slide (strict)"("Visible"=TRUE, "Scale.Maximum"=100.0 ("Scale.Range:Maximum")) -> ()  [unwired: 2 in, 2 out]
                n207 = property on="Test Ring" class="Ring (strict)"("Visible"=FALSE) -> ()  [unwired: 2 in, 2 out]
              }
            }
          }
        }
        n208 = property on="Progress" class="Clust (strict)"("Visible"=FALSE) -> ()  [unwired: 2 in, 2 out]
      }
      event "Test Name": Mouse Enter {
        # "Populate the ring with the list of tests"
        n209 = event-data() -> ()  [unwired: 1 in, 1 out]
        n210 = call <vilib>:"NT Read String Array.vi"("Name"="/TestMode/TestList") -> ("String Array"=w344:string[])  [unwired: 9 in, 1 out]
        n211 = Build Array (concatenate)("Select the test to run...", w344) -> (w343:string[])
        n212 = property on="Test Name" class="Ring (strict)"("Strings []"=w343) -> ()  [unwired: 2 in, 2 out]
      }
      event "Test Name": Value Change {
        w346 = FALSE ("Visible")
        # "Tell the robot the test name to run"
        n213 = event-data() -> ("NewVal"=w350:u16)  [unwired: 1 in]
        n214 = property on="Test Name" class="Ring (strict)"() -> ("Strings []"=w351:string[])  [unwired: 2 in, 2 out]
        n215 = local write "Progress"(T6 {"Test Progress"=0, "Test Progress Text"=""} ("Progress")) -> ()
        n216 = Index Array(array=w351, index=w350) -> (element=w349:string)
        n217 = call <vilib>:"NT Write String.vi"("String"=w349, "Name"="/TestMode/TestName") -> ()  [unwired: 9 in, 1 out]
        n218 = property on="Progress" class="Clust (strict)"("Visible"=TRUE) -> ()  [unwired: 2 in, 2 out]
        n219 = property on="Motor" class="Clust (strict)"("Visible"=w346) -> ()  [unwired: 2 in, 2 out]
        n220 = property on="Test Slider" class="Slide (strict)"("Visible"=w346) -> ()  [unwired: 2 in, 2 out]
        n221 = property on="On/Off" class="Bool (strict)"("Visible"=w346) -> ()  [unwired: 2 in, 2 out]
        n222 = property on="Rev/Fwd" class="Clust (strict)"("Visible"=w346) -> ()  [unwired: 2 in, 2 out]
        n223 = property on="Test Ring" class="Ring (strict)"("Visible"=w346) -> ()  [unwired: 2 in, 2 out]
      }
      event "Select Auto": Mouse Enter {
        # "Populate the combo box with the list of autonomous options"
        n224 = event-data() -> ()  [unwired: 1 in, 1 out]
        n225 = call <vilib>:"NT Read String Array.vi"("Name"="Auto List") -> ("String Array"=w353:string[])  [unwired: 9 in, 1 out]
        n226 = property on="Select Auto" class="CmbBox"("Strings[]"=w353) -> ()  [unwired: 2 in, 2 out]
      }
      event "Select Auto": Value Change {
        # "User modified the Auto Selection. Write to NT variable so robot knows."
        n227 = event-data() -> ("NewVal"=w356:string)  [unwired: 1 in]
        n228 = call <vilib>:"NT Write String.vi"("String"=w356, "Name"="Auto Selector") -> ()  [unwired: 9 in, 1 out]
      }
      event "Command Selection": Value Change {
        # "Get the params and show in table"
        n229 = event-data() -> ("NewVal"=w362:i32)  [unwired: 1 in]
        n230 = property on="Command Selection" class="MCListbox (strict)"() -> ("ItemNames"=w360:string[][])  [unwired: 2 in, 2 out]
        n231 = call <vilib>:"WPI_DashboardUpdate Command Params.vi"("NewVal"=w362, "Commands"=w360, "Param Tbl"=w361) -> ()  [unwired: 8 in, 1 out]
      }
      event "Execute Command": Value Change {
        # "Started one, Unique ID holds\nresponse"
        n232 = event-data() -> ()  [unwired: 1 in, 1 out]
        n233 = property on="Command Selection" class="MCListbox (strict)"() -> ("ItemNames"=w373:string[][])  [unwired: 2 in, 2 out]
        n234 = Index Array(array=w373, index (row)="Command Selection", index (col)=0) -> (element=w371:string)
        n235 = call <vilib>:"Invoke Commands.vi"("Command Params"="Command Params", "Function Name"=w371) -> ("Params"=w367:u8, "Started"=w366:bool)  [unwired: 7 in, 1 out]
        n236 = Array Subset(array="Command Params", length (row)=w367) -> (w368:string[][])  [unwired: 3 in]
        n237 = Select(t="Executing" ("Cmd Status"), s=w366, f="" ("Cmd Status")) -> (s? t:f=→"Cmd Status":string)
      }
      event "Command Selection": Double Click {
        n238 = event-data() -> ("Row"=w381:i32)  [unwired: 1 in]
        n239 = property on="Command Selection" class="MCListbox (strict)"() -> ("ItemNames"=w384:string[][])  [unwired: 2 in, 2 out]
        n240 = local read "Command Params"() -> (w380:string[][])
        n241 = Index Array(array=w384, index (row)=w381, index (col)=0) -> (element=w382:string)
        n242 = call <vilib>:"Invoke Commands.vi"("Command Params"=w380, "Function Name"=w382) -> ("Params"=w379:u8, "Started"=w374:bool)  [unwired: 7 in, 1 out]
        n243 = Array Subset(array=w380, length (row)=w379) -> (w378:string[][])  [unwired: 3 in]
        n244 = Select(t="Executing" ("Cmd Status"), s=w374, f="" ("Cmd Status")) -> (s? t:f=w375:string)
        n245 = local write "Cmd Status"(w375) -> ()
      }
      event "CheckList": Double Click {
        # "Shift clears all"
        # "Update symbols on the listbox"
        n246 = event-data() -> ("PlatMods.Shift"=w386:bool, "Row"=w388:i32)  [unwired: 1 in]
        n247 = case shown="True" w386 {
          tunnel: w388 -> [w392 _]
          tunnel: 1 -> [w391 _]
          frame False {
            n248 = property on="CheckList" class="LstBox (strict)"() -> ("Item Symbols"=w390:i32[])  [unwired: 2 in, 2 out]
            n249 = Replace Array Subset(array=w390, new element=w391, index=w392) -> (w389:i32[])
            n250 = property on="CheckList" class="LstBox (strict)"("Item Symbols"=w389) -> ()  [unwired: 2 in, 2 out]
          }
          frame True {
            w393 = 0 ("Top Row")
            n251 = property on="CheckList" class="LstBox (strict)"() -> ("Number of Rows"=w395:u32)  [unwired: 2 in, 2 out]
            n252 = Initialize Array(0, w395) -> (w394:i32[])
            n253 = property on="CheckList" class="LstBox (strict)"("Top Row"=w393, "Value"=w393, "Item Symbols"=w394) -> ()  [unwired: 2 in, 2 out]
          }
        }
      }
      event "CheckList": Key Down {
        # "Update symbols on the listbox\nLeft and right keys check and uncheck"
        n254 = event-data() -> ("VKey"=w399:T19)  [unwired: 1 in]
        n255 = case shown="\"Left\", \"Right\"" w399 {
          selector: w399 -> [w404 _]
          tunnel: eventvkey."Left" ("VKey") -> [w402 _]
          frame "Left", "Right" {
            n256 = Equal?(x=w402, y=w404) -> (x = y?=w403:bool)
            n257 = Select(t=0, s=w403, f=1) -> (s? t:f=w405:i32)
            n258 = property on="CheckList" class="LstBox (strict)"() -> ("Item Symbols"=w408:i32[])  [unwired: 2 in, 2 out]
            n259 = Replace Array Subset(array=w408, new element=w405, index="CheckList") -> (w407:i32[])
            n260 = property on="CheckList" class="LstBox (strict)"("Item Symbols"=w407) -> ()  [unwired: 2 in, 2 out]
          }
          frame Default {
          }
        }
      }
      event "Motor.Enable": Value Change {
        # "When the test mode otor enable helper is set, update that\ntree row item's value"
        n261 = event-data() -> ("NewVal"=w414:bool)  [unwired: 1 in]
        n262 = Unbundle("Motor") -> ("Value"=w413:dbl)  [unwired: 1 out]
        n263 = Select(t=w413, s=w414, f=0.0) -> (s? t:f=w411:dbl)
        n264 = call <vilib>:"NT Write Number.vi"("Numeric"=w411, "Name"=w410) -> ()  [unwired: 9 in, 1 out]
      }
      event "Test Slider": Value Change {
        # "When the test mode slider helper is set, update that\ntree row item's value"
        n265 = event-data() -> ("NewVal"=w417:dbl)  [unwired: 1 in]
        n266 = call <vilib>:"NT Write Number.vi"("Numeric"=w417, "Name"=w418) -> ()  [unwired: 9 in, 1 out]
      }
      event "On/Off": Value Change {
        # "When the test mode on/off helper value is set, update that\ntree row item's value"
        n267 = event-data() -> ("NewVal"=w422:bool)  [unwired: 1 in]
        n268 = Boolean To (0,1)(Boolean=w422) -> (0, 1=w421:i16)
        n269 = call <vilib>:"NT Write Number.vi"("Numeric"=w421, "Name"=w420) -> ()  [unwired: 9 in, 1 out]
      }
      event "Rev/Fwd": Value Change {
        # "When the test mode helper value for relays is set, update that\ntree row item's value"
        n270 = event-data() -> ("NewVal.Forward"=w430:bool, "NewVal.Reverse"=w429:bool)  [unwired: 1 in]
        n271 = Boolean To (0,1)(Boolean=w430) -> (0, 1=w426:i16)
        n272 = Boolean To (0,1)(Boolean=w429) -> (0, 1=w428:i16)
        n273 = Negate(x=w428) -> (-x=w427:i16)
        n274 = Add(x=w426, y=w427) -> (x+y=w425:i16)
        n275 = call <vilib>:"NT Write Number.vi"("Numeric"=w425, "Name"=w424) -> ()  [unwired: 9 in, 1 out]
      }
      event "Test Ring": Value Change {
        # "When a test mode helper value is selected from the ring,\nset the tree item's variable to the string value"
        n276 = event-data() -> ("NewVal"=w434:u16)  [unwired: 1 in]
        n277 = property on="Test Ring" class="Ring (strict)"() -> ("Strings []"=w435:string[])  [unwired: 2 in, 2 out]
        n278 = Index Array(array=w435, index=w434) -> (element=w433:string)
        n279 = call <vilib>:"NT Write String.vi"("String"=w433, "Name"=w432) -> ()  [unwired: 9 in, 1 out]
      }
      event "Rec Mode": Value Change {
        # "Update globals for recording mode and path to read log from.\nClear when logging and let NetworkTables set path for vision to\nuse."
        n280 = event-data() -> ("NewVal"=w446:enum32{"Stop", "Record", "Playback"})  [unwired: 1 in]
        n281 = global write "WPI_DashboardLogging Global.vi" "Logging Filename"(path "") -> ()
        n282 = global write "WPI_DashboardLogging Global.vi" "Recording"(w446) -> ()
        n283 = case shown="\"Playback\"" w446 {
          tunnel: w445 -> [_ w448 w457]
          tunnel: [_ _ w456] -> w443
          tunnel: [_ _ w455] -> _
          tunnel: w441 -> [_ _ w453]
          tunnel: cluster{i32, i32} {-250, 170} -> [_ _ w452]
          tunnel: [_ _ T20 {"Image Size"=TRUE, "Image Type"=TRUE, "Pixel Value"=TRUE, "ROI Information"=TRUE, "Zoom Factor"=FALSE} ("Image Information Shown:All Elements")] -> w439
          tunnel: [_ _ TRUE ("Zoom Factor")] -> w438
          tunnel: w437 -> [_ _ w449]
          frame Default {
          }
          frame "Stop", "Record" {
            # "Place Window too"
            n284 = invoke class="VI" method="FP.Close"(reference=w448) -> (reference out=w447:refnum<vi>)  [unwired: 2 in, 2 out]
            n285 = invoke class="VI" method="Abort VI"(reference=w447) -> ()  [unwired: 2 in, 3 out]
          }
          frame "Playback" {
            n286 = call "Open Playback Panel.vi"("Offset"=w452, "DB VI Ref"=w453, "Playback in"=w457) -> ("Playback out"=w454:refnum<vi>)  [unwired: 8 in]
            n287 = register-events(w454, w449) -> (reference out=w456:refnum<event-registration>, error out=w455:errorcluster)  [unwired: 2 in]
          }
        }
        n288 = property on="Camera Image" class="ImageControl"("Image Information Shown"=w439, "Image Information Visible"=w438) -> ()  [unwired: 2 in, 2 out]
        n289 = call <vilib>:"WPI_DashboardNT Log FieldName Cache.vi"("Operation"=enum16{"Lookup/Add", "Index", "Clear"}."Clear") -> ()  [unwired: 8 in, 3 out]
      }
      event Panel Close {
        w459 = enum32{"Stop", "Record", "Playback"}."Stop" ("Rec Mode")
        # "Playback window has been closed, abort"
        n290 = event-data() -> ()  [unwired: 1 in, 4 out]
        n291 = local write "Rec Mode"(w459) -> ()
        n292 = global write "WPI_DashboardLogging Global.vi" "Recording"(w459) -> ()
      }
      event Panel Close {
        # "Abort playback window and ourself"
        n293 = event-data() -> ()  [unwired: 1 in, 4 out]
        n294 = invoke class="VI" method="FP.Close"(reference=w463) -> (reference out=w462:refnum<vi>)  [unwired: 2 in, 2 out]
        n295 = invoke class="VI" method="Abort VI"(reference=w462) -> (error out=w461:errorcluster)  [unwired: 2 in, 2 out]
        n296 = invoke class="VI" method="Abort VI"(error in=w461) -> ()  [unwired: 2 in, 3 out]
      }
      event User Event {
        n297 = event-data() -> ("IDs"=w470:cluster{"RPC field ID":u16, "Unique ID":u16}, "String"=w469:string)  [unwired: 1 in]
        n298 = Bundle("IDs"=w470, "String"=w469) -> (w468:T8)  [unwired: 1 in]
        n299 = call <vilib>:"Retrieve RPC Response.vi"("RPC Response"=w468) -> ("Output"=w466:string[][])  [unwired: 10 in]
        n300 = Build Array (concatenate)(w464, w466) -> (w465:string[][])
        n301 = local write "Command Params"(w465) -> ()
        n302 = local write "Cmd Status"("" ("Cmd Status")) -> ()
      }
      event "Tree": Double Click {
        n303 = event-data() -> ("PlatMods"=w474:T23, "Tag"=w473:string)  [unwired: 1 in]
        n304 = Unbundle(w474) -> ("Shift"=w472:bool)  [unwired: 4 out]
        n305 = Not(x=w472) -> (.not. x?=w471:bool)
        n306 = call <vilib>:"NT Update Persistence.vi"("Persistence"=w471, "Name"=w473) -> ()  [unwired: 9 in, 1 out]
      }
    }
  }
  n307 = while {
    tunnel: w69 -> [w477]
    i -> [w480]
    stop <- FALSE stop-if-true
    n308 = Wait (ms)(milliseconds to wait=u32 100) -> ()  [unwired: 1 out]
    n309 = case shown="\"Playback\"" "Rec Mode" {
      tunnel: w480 -> [_ _ w495]
      tunnel: [u32 2829099 ("Base Color") u32 11141120 ("Target Color") w484] -> w476
      frame "Stop", Default {
        # "Reset the color, extra updates don't cost much"
      }
      frame "Record" {
      }
      frame "Playback" {
        # "Playback"
        n310 = Quotient & Remainder(x=w495, y=u32 50 ("milliseconds to wait")) -> (x-y*floor(x/y)=w491:u32)  [unwired: 1 out]
        n311 = Divide(x=w491, y=u32 50 ("milliseconds to wait")) -> (x/y=w488:dbl)
        n312 = Multiply(x=6.283185307179586, y=w488) -> (x*y=w493:dbl)
        n313 = Sine(x=w493) -> (sin(x)=w492:dbl)
        n314 = Absolute Value(x=w492) -> (abs(x)=w485:dbl)
        n315 = call "Interpolate RGB Color.vi"("Proportion"=w485, "Target Color"=u32 30976, "Base Color"=u32 2829099) -> ("Result Color"=w484:u32)  [unwired: 8 in]
      }
    }
    n316 = property class="Pane"(reference=w477, "PaneColor"=w476) -> ()  [unwired: 1 in, 2 out]
  }
  n317 = local write "Dashboard Tab"(T2."Drive" ("Dashboard Tab")) -> ()
  n318 = property on="On/Off" class="Bool (strict)"("Visible"=w38) -> ()  [unwired: 2 in, 2 out]
  n319 = property on="Motor" class="Clust (strict)"("Visible"=w38) -> ()  [unwired: 2 in, 2 out]
  n320 = property on="Progress" class="Clust (strict)"("Visible"=w38) -> ()  [unwired: 2 in, 2 out]
  n321 = property on="Test Ring" class="Ring (strict)"("Visible"=w38) -> ()  [unwired: 2 in, 2 out]
  n322 = property on="Rev/Fwd" class="Clust (strict)"("Visible"=w38) -> ()  [unwired: 2 in, 2 out]
  n323 = while {
    tunnel: u16 1741 ("timeout ms (25000)") -> [w497]
    stop <- FALSE stop-if-true
    n324 = TCP Create Listener(10:w497) -> (0:w496:errorcluster, 3:w498:refnum<k5>)  [unwired: 4 in, 1 out]
    n325 = case shown="No Error" w496 {
      selector: w496 -> [w500 _]
      tunnel: w498 -> [w501 _]
      frame No Error {
        n326 = while {
          tunnel: w501 -> [w504]
          tunnel: w500 -> [w503]
          stop <- FALSE stop-if-true
          n327 = TCP Wait On Listener(8:w503, 11:w504) -> (0:w505:errorcluster, 4:w506:refnum<k5>)  [unwired: 2 in, 3 out]
          n328 = local write "TCP"(w506) -> ()
          n329 = case shown="No Error" w505 {
            frame No Error {
            }
            frame Error {
              n330 = Wait (ms)(milliseconds to wait=u32 1000) -> ()  [unwired: 1 out]
            }
          }
        }
      }
      frame Error {
        n331 = Wait (ms)(milliseconds to wait=u32 1000) -> ()  [unwired: 1 out]
      }
    }
  }
  n332 = local write "Command Selection"(u16 0 ("milliseconds to wait")) -> ()
  n333 = local write "Command Params"(string[][] [] ("Command Params")) -> ()
  n334 = global write "WPI_DashboardLogging Global.vi" "Recording"(w63) -> ()
  n335 = local write "Rec Mode"(w63) -> ()
  n336 = call <vilib>:"NT Write String.vi"("String"="Select Auto", "Name"="Auto Selector") -> ()  [unwired: 9 in, 1 out]
  n337 = call-poly "VISA Configure Serial Port"("VISA resource name"=refnum<visa-resource-name> "COM3", "baud rate (9600)"=u32 9600, "data bits (8)"=u16 8) -> ("VISA resource name out"=w4:refnum<visa-resource-name>)  [unwired: 11 in, 1 out]
  n338 = while {
    tunnel: w4 -> [w511]
    tunnel: [w510] -> w3
    stop <- FALSE stop-if-true
    n339 = VISA Read(VISA resource name=w511, byte count=u32 1) -> (VISA resource name out=w510:refnum<visa-resource-name>, read buffer=w512:string)  [unwired: 1 in, 2 out]
    "read buffer" <- w512
    n340 = call-poly <vilib>:"NT Write Value.vi"("String"=w512, "Name"="Fire") -> ()  [unwired: 9 in, 1 out]
  }
  n341 = VISA Close(VISA resource name=w3) -> ()  [unwired: 1 in, 1 out]
